vi "Joules to FE.vi"(5 "J":dbl) -> (2 "FE":dbl)   [LabVIEW 2023]
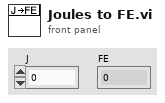
[diagram p1: front panel]
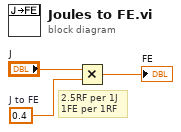
[diagram p0: block diagram]
diagram:
  w3 = 0.4  # J to FE
  # "2.5RF per 1J\n1FE per 1RF"
  n1 = Multiply(x="J", y=w3) -> (x*y=→"FE":dbl)
